vi "ROI_define_mosaic.vi"(4 "FOV size (um)":dbl=200.0 min=0.0 step=0.1 format="%#.1f", 6 "error in":errorcluster, 7 "Mosaic size Y":i32(ring) items=["1", "3", "5"], 8 "Mosaic size X":i32(ring) items=["1", "3", "5"], 9 "XY positions IN":dbl[][](array[numeric])) -> (0 "error out":errorcluster, 5 "XY positions OUT":dbl[][](array[numeric]))   [LabVIEW 2015]
uses:
  GLOBAL/Global_ASI_stage.vi
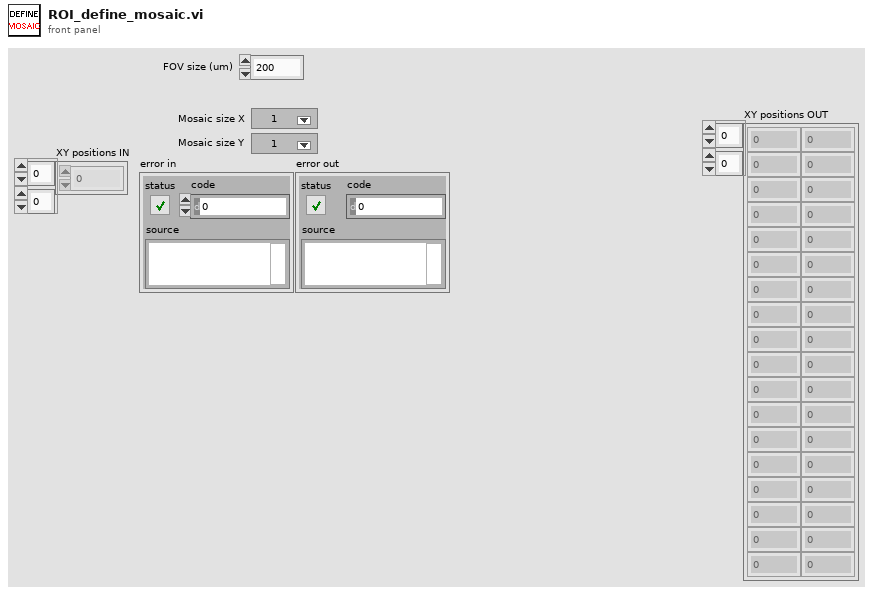
[diagram p1: front panel]
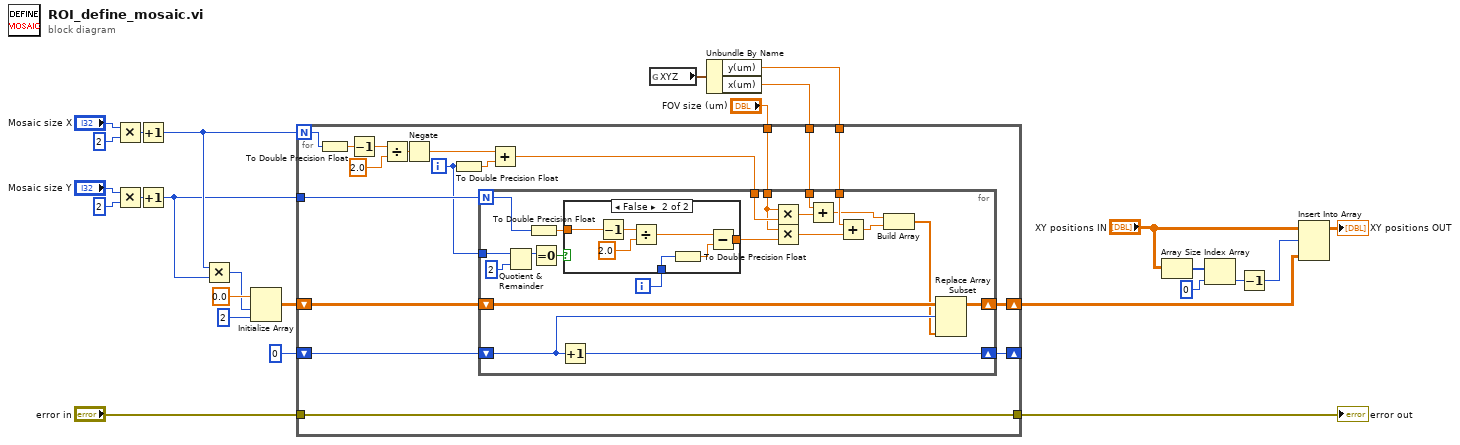
[diagram p0: block diagram]
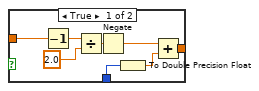
[diagram p2: hidden frame]
diagram:
  n1 = Multiply(x="Mosaic size X", y=2) -> (x*y=w20:i32)
  n2 = Multiply(x="Mosaic size Y", y=2) -> (x*y=w15:i32)
  n3 = Increment(x=w20) -> (x+1=w19:i32)
  n4 = Increment(x=w15) -> (x+1=w16:i32)
  n5 = Multiply(x=w19, y=w16) -> (x*y=w24:i32)
  n6 = Initialize Array(0.0 ("element"), w24, 2 ("dimension size")) -> (w23:dbl[][])
  n7 = global read "Global_ASI_stage.vi" "XYZ"() -> (w13:cluster{"x(um)":dbl, "y(um)":dbl, "z(um)":dbl})
  n8 = Unbundle By Name(w13) -> ("y(um)"=w11:dbl, "x(um)"=w12:dbl)
  n9 = for {
    N: w19 -> [w38]
    tunnel: w16 -> [w40]
    shift-right: [w36] -> w6
    shift-left: w23 -> [w37]
    shift-right: [w34] -> _
    shift-left: 0 ("dimension size") -> [w35]
    tunnel: "FOV size (um)" -> [w33]
    tunnel: w12 -> [w30]
    tunnel: w11 -> [w29]
    tunnel: "error in" -> [w28]
    tunnel: [w28] -> w2
    i -> [w27]
    n10 = To Double Precision Float(number=w38) -> (double precision float=w41:dbl)
    n11 = Decrement(x=w41) -> (x-1=w44:dbl)
    n12 = Divide(x=w44, y=2.0) -> (x/y=w32:dbl)
    n13 = Negate(x=w32) -> (-x=w42:dbl)
    n14 = To Double Precision Float(number=w27) -> (double precision float=w31:dbl)
    n15 = Add(x=w42, y=w31) -> (x+y=w39:dbl)
    n16 = for {
      N: w40 -> [w50]
      tunnel: w39 -> [w60]
      shift-right: [w64] -> w36
      shift-left: w37 -> [w63]
      shift-right: [w61] -> w34
      shift-left: w35 -> [w62]
      tunnel: w33 -> [w58]
      tunnel: w30 -> [w56]
      tunnel: w29 -> [w54]
      tunnel: w27 -> [w45]
      i -> [w46]
      n17 = Quotient & Remainder(x=w45, y=2) -> (x-y*floor(x/y)=w48:i32)  [unwired: 1 out]
      n18 = To Double Precision Float(number=w50) -> (double precision float=w65:dbl)
      n19 = Equal To 0?(x=w48) -> (x = 0?=w47:bool)
      n20 = Increment(x=w62) -> (x+1=w61:i32)
      n21 = case shown="False" w47 {
        tunnel: w65 -> [w73 w80]
        tunnel: w46 -> [w69 w77]
        tunnel: [w68 w76] -> w59
        frame True {
          n22 = Decrement(x=w73) -> (x-1=w70:dbl)
          n23 = Divide(x=w70, y=2.0) -> (x/y=w67:dbl)
          n24 = Negate(x=w67) -> (-x=w72:dbl)
          n25 = To Double Precision Float(number=w69) -> (double precision float=w66:dbl)
          n26 = Add(x=w72, y=w66) -> (x+y=w68:dbl)
        }
        frame False {
          n27 = Decrement(x=w80) -> (x-1=w78:dbl)
          n28 = Divide(x=w78, y=2.0) -> (x/y=w74:dbl)
          n29 = To Double Precision Float(number=w77) -> (double precision float=w75:dbl)
          n30 = Subtract(x=w74, y=w75) -> (x-y=w76:dbl)
        }
      }
      n31 = Multiply(x=w58, y=w60) -> (x*y=w57:dbl)
      n32 = Multiply(x=w58, y=w59) -> (x*y=w55:dbl)
      n33 = Add(x=w56, y=w57) -> (x+y=w53:dbl)
      n34 = Add(x=w54, y=w55) -> (x+y=w52:dbl)
      n35 = Build Array(w53, w52) -> (w51:dbl[])
      n36 = Replace Array Subset(array=w63, new element=w51, index (row)=w62) -> (w64:dbl[][])  [unwired: 1 in]
    }
  }
  "error out" <- w2
  n37 = Array Size(array="XY positions IN") -> (size(s)=w10:i32[])
  n38 = Index Array(array=w10, index=0) -> (element=w8:i32)
  n39 = Decrement(x=w8) -> (x-1=w7:i32)
  n40 = Insert Into Array(array="XY positions IN", index (row)=w7, new element=w6) -> (→"XY positions OUT":dbl[][])  [unwired: 1 in]
